vi "scanraw.vi"(5 "Offset":u16(ring)=174 items=["tinySA"=128, "tinySA_Ultra"=174], 7 "Points":u32=450, 8 "Error in":errorcluster, 9 "Stop (Hz)":u32=100000000 format="%.0p", 10 "Start (Hz)":u32 format="%.0p", 11 "VISA name in":refnum<visa-resource-name>) -> (0 "Error out":errorcluster, 2 "Power (dBm)":dbl[](graph), 3 "VISA name out":refnum<visa-resource-name>)   [LabVIEW 2012]
panel:
  out "extracted record":string
  out "cmd echo":string
  out "i":i32
  out "response":string
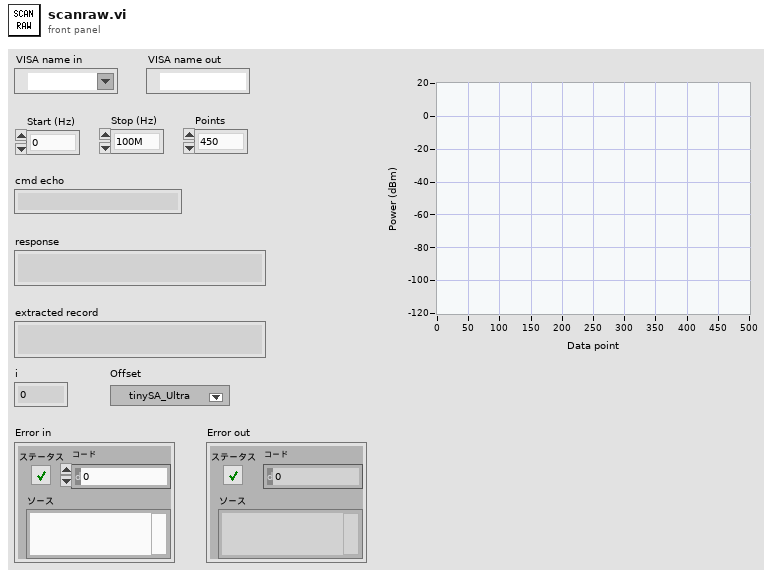
[diagram p1: front panel]
types:
  T1 = enum16{"big-endian, network order", "native, host order", "little-endian"}
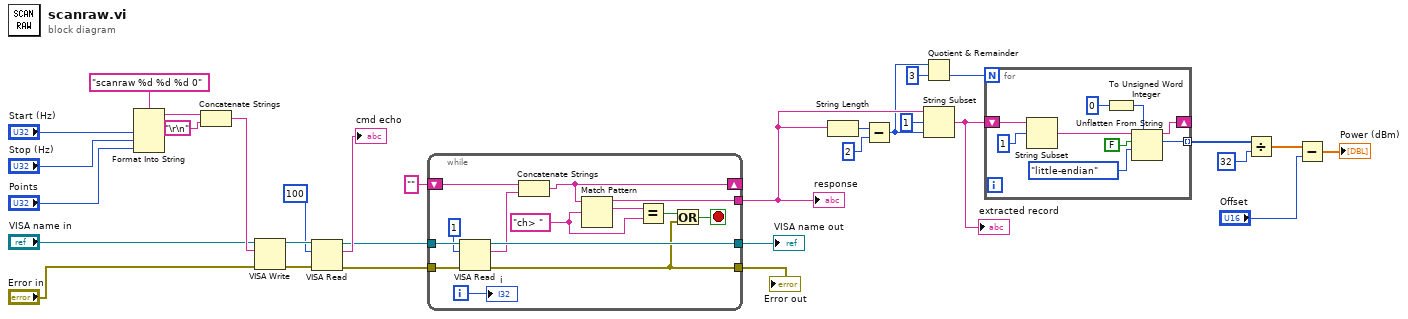
[diagram p0: block diagram]
diagram:
  n1 = Format Into String(format string="scanraw %d %d %d 0" ("形式文字列"), "Start (Hz)", "Stop (Hz)", "Points") -> (resulting string=w8:string)  [unwired: 2 in, 1 out]
  n2 = Concatenate Strings(w8, "\r\n") -> (w30:string)
  n3 = VISA Write(VISA resource name="VISA name in", write buffer=w30, error in (no error)="Error in") -> (VISA resource name out=w27:refnum<visa-resource-name>, error out=w26:errorcluster)  [unwired: 1 out]
  n4 = VISA Read(VISA resource name=w27, byte count=u32 100 ("バイトカウント"), error in (no error)=w26) -> (VISA resource name out=w22:refnum<visa-resource-name>, read buffer=→"cmd echo":string, error out=w21:errorcluster)  [unwired: 1 out]
  n5 = while {
    shift-right: [w39] -> _
    shift-left: "" -> [w40]
    tunnel: [w38] -> w23
    tunnel: w22 -> [w45]
    tunnel: [w42] -> w7
    tunnel: w21 -> [w44]
    tunnel: [w32] -> w6
    i -> [w35]
    stop <- w34 stop-if-true
    w36 = "ch> " ("正規表現")
    n6 = VISA Read(VISA resource name=w45, byte count=u32 1 ("バイトカウント"), error in (no error)=w44) -> (VISA resource name out=w42:refnum<visa-resource-name>, read buffer=w41:string, error out=w32:errorcluster)  [unwired: 1 out]
    n7 = Concatenate Strings(w40, w41) -> (w39:string)
    n8 = Match Pattern(string=w39, regular expression=w36) -> (before substring=w38:string, match substring=w37:string)  [unwired: 1 in, 2 out]
    n9 = Equal?(x=w37, y=w36) -> (x = y?=w33:bool)
    n10 = Or(x=w33, y=w32) -> (x .or. y?=w34:bool)
    "i" <- w35
  }
  "response" <- w23
  "VISA name out" <- w7
  "Error out" <- w6
  n11 = String Length(string=w23) -> (length=w20:i32)
  n12 = Subtract(x=w20, y=2) -> (x-y=w11:i32)
  n13 = Quotient & Remainder(x=w11, y=3) -> (floor(x/y)=w12:i32)  [unwired: 1 out]
  n14 = String Subset(string=w23, offset (0)=1 ("オフセット (0)"), length (rest)=w11) -> (substring=w16:string)
  "extracted record" <- w16
  n15 = for {
    N: w12 -> [_]
    shift-right: [w51] -> _
    shift-left: w16 -> [w47]
    tunnel: [w50] -> w15 mode=indexing
    n16 = String Subset(string=w47, offset (0)=1 ("オフセット (0)")) -> (substring=w46:string)  [unwired: 1 in]
    n17 = To Unsigned Word Integer(number=u16 0 ("数値")) -> (unsigned 16bit integer=w54:u16)
    n18 = Unflatten From String(type=w54, binary string=w46, data includes array or string size? (T)=FALSE ("データは配列または文字列サイズを含む? (T)"), byte order (0:big-endian, network order)=T1."little-endian" ("バイト順序 (0:ビッグエンディアン、ネットワーク順)")) -> (rest of the binary string=w51:string, value=w50:u16)  [unwired: 1 in, 1 out]
  }
  n19 = Divide(x=w15, y=32) -> (x/y=w13:dbl[])
  n20 = Subtract(x=w13, y="Offset") -> (x-y=→"Power (dBm)":dbl[])
